vi "_FPGA_AuxVoltage.vi"(5 "Cycle in":u64, 7 "MaxCycle-1 in":u32=1, 8 "Cycle 2":u32=2147483648, 9 "Voltage2":fxp<+/-,16,14>, 10 "Cycle 1":u32=2147483648, 11 "Voltage1":fxp<+/-,16,14>) -> (1 "AuxVoltage":fxp<+/-,16,14>)   [LabVIEW 2018]
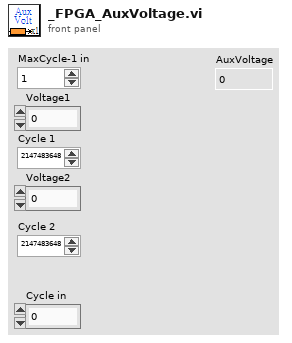
[diagram p1: front panel]
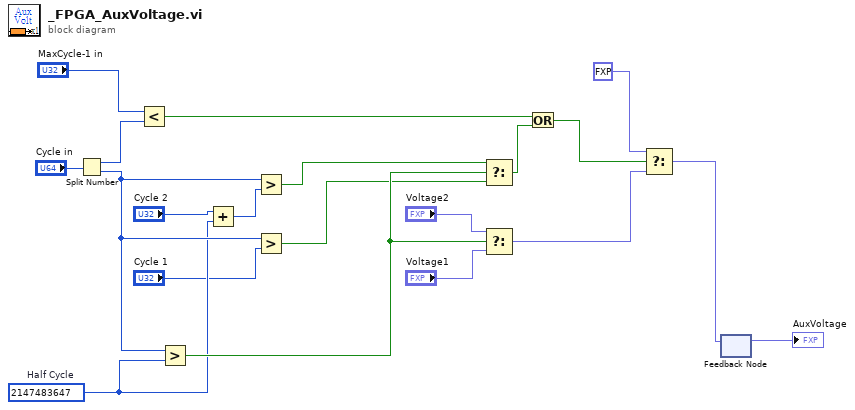
[diagram p0: block diagram]
diagram:
  w6 = u32 2147483647  # Half Cycle
  n1 = Split Number(x="Cycle in") -> (hi(x)=w19:u32, lo(x)=w14:u32)
  n2 = Less?(x="MaxCycle-1 in", y=w19) -> (x < y?=w18:bool)
  n3 = Greater?(x=w14, y=w6) -> (0:w13:bool)
  n4 = Add(x="Cycle 2", y=w6) -> (x+y=w4:u32)
  n5 = Greater?(x=w14, y=w4) -> (0:w12:bool)
  n6 = Greater?(x=w14, y="Cycle 1") -> (0:w11:bool)
  n7 = Select(t=w12, s=w13, f=w11) -> (s? t:f=w10:bool)
  n8 = Select(t="Voltage2", s=w13, f="Voltage1") -> (s? t:f=w2:fxp<+/-,16,14>)
  n9 = Or(x=w18, y=w10) -> (x .or. y?=w3:bool)
  n10 = Select(t=fxp<+/-,16,14> 0.0, s=w3, f=w2) -> (s? t:f=w17:fxp<+/-,16,14>)
  n11 = feedback-in #1(w17) -> ()
  n12 = feedback #1() -> (→"AuxVoltage":fxp<+/-,16,14>)  [unwired: 1 in]
